vi "Plugin Configuration.Create.vi"(8 "error in (no error)":errorcluster, 10 "Plugin Configuration cluster":T1={"name"="", "class"="", "cycle timing"={"priority"=0, "decimation"=1, "offset"=0}, "Transfer Groups"=[], "settings"=[]}, 11 "Plugin Configuration in":refnum<class "Plugin Configuration.lvclass">) -> (0 "error out":errorcluster, 3 "Plugin Configuration out":refnum<class "Plugin Configuration.lvclass">)   [LabVIEW 2017, in "DSF Core.lvlib" / "Plugin Configuration.lvclass"]
uses:
  Plugin Configuration.lvclass
  DSF Configuration API/Public/Controls/DSF Engine Plugin Configuration.ctl
  DSF Configuration API/Public/Controls/DSF Timing Info.ctl
  DSF Configuration API/Public/Controls/DSF Engine Transfer Group Configuration.ctl
  DSF Configuration API/Public/Controls/DSF Direction.ctl
  DSF Configuration API/Public/Controls/DSF Engine Transfer Configuration.ctl
  DSF Configuration API/Public/Controls/DSF Byte Order.ctl
  DSF Configuration API/Public/Controls/DSF Engine Channel Configuration.ctl
  DSF Configuration API/Public/Controls/DSF Data Type.ctl
  DSF Configuration API/Public/Controls/DSF Settings Info.ctl
  Transfer Group/Transfer Group Configuration.lvclass
  Plugin Configuration.lvclass/Plugin Configuration.ctl
  DSF Core.lvlib
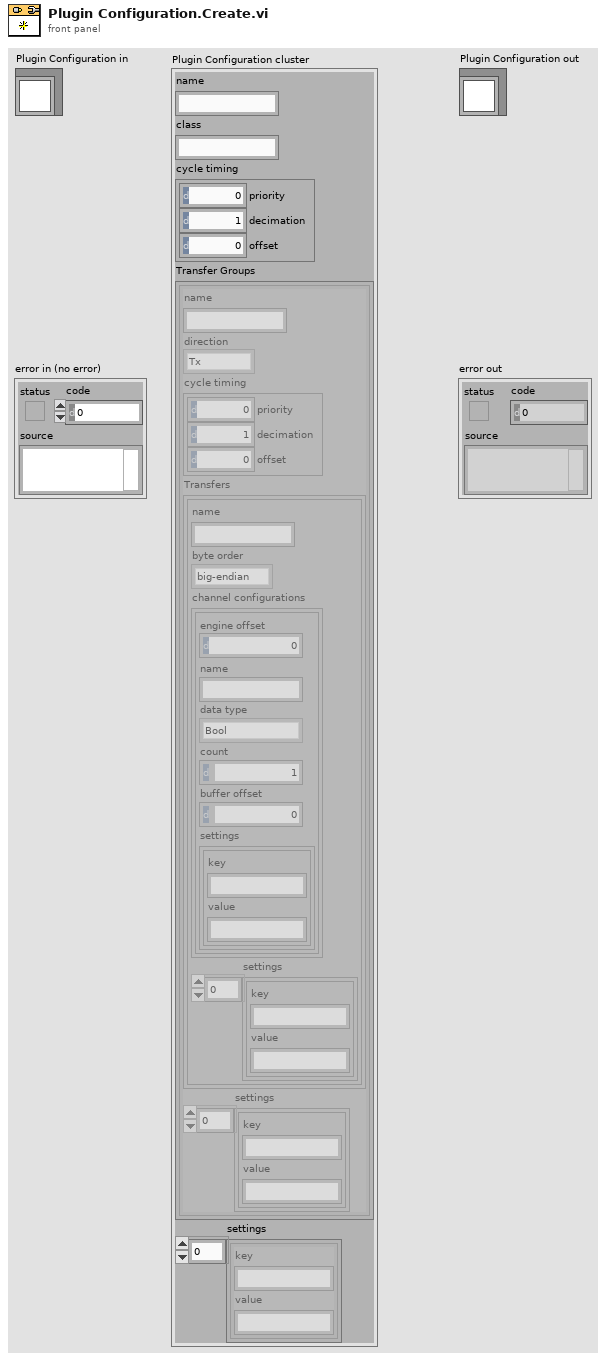
[diagram p1: front panel]
types:
  T1 = typedef "DSF Core.lvlib/DSF Engine Plugin Configuration.ctl" = cluster{"name":string, "class":string, "cycle timing":T2, "Transfer Groups":T3[], "settings":T9}
  T2 = typedef "DSF Core.lvlib/DSF Timing Info.ctl" = cluster{"priority":u64, "decimation":u64, "offset":u64}
  T3 = typedef "DSF Core.lvlib/DSF Engine Transfer Group Configuration.ctl" = cluster{"name":string, "direction":T4, "cycle timing":T2, "Transfers":T5[], "settings":T9}
  T4 = typedef "DSF Core.lvlib/DSF Direction.ctl" = enum8{"Tx", "Rx"}
  T5 = typedef "DSF Core.lvlib/DSF Engine Transfer Configuration.ctl" = cluster{"name":string, "byte order":T6, "channel configurations":T7[], "settings":T9}
  T6 = typedef "DSF Core.lvlib/DSF Byte Order.ctl" = enum8{"big-endian", "little-endian"}
  T7 = typedef "DSF Core.lvlib/DSF Engine Channel Configuration.ctl" = cluster{"engine offset":u64, "name":string, "data type":T8, "count":u64, "buffer offset":u64, "settings":T9}
  T8 = typedef "DSF Core.lvlib/DSF Data Type.ctl" = enum8{"Bool", "SGL", "DBL", "I8", "I16", "I32", "I64", "U8", "U16", "U32", "U64"}
  T9 = typedef "DSF Core.lvlib/DSF Settings Info.ctl" = cluster{"key":string, "value":string}[]
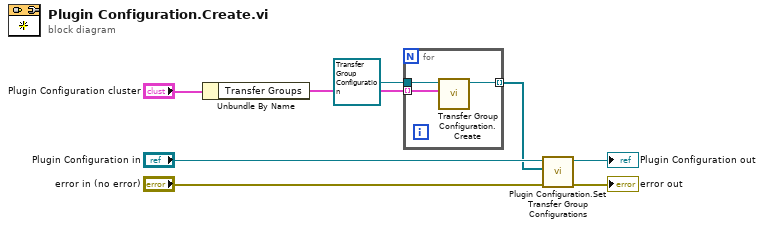
[diagram p0: block diagram]
diagram:
  n1 = Unbundle By Name("Plugin Configuration cluster") -> ("Transfer Groups"=w3:T3[])
  n2 = for {
    tunnel: w3 -> [w10] mode=indexing
    tunnel: refnum<class "Transfer Group Configuration.lvclass"> refnum ("DSF.Shared.lvlib:Transfer Group Configuration") -> [w9]
    tunnel: [w8] -> w1 mode=indexing
    n3 = call "Transfer Group Configuration.Create.vi"("Transfer Group Configuration"=w10, "Transfer Group Configuration in"=w9) -> ("Transfer Group Configuration out"=w8:refnum<class "Transfer Group Configuration.lvclass">)  [unwired: 8 in, 1 out]
  }
  n4 = call "Plugin Configuration.Set Transfer Group Configurations.vi"("Transfer Group Configurations"=w1, "Plugin Configuration in"="Plugin Configuration in") -> ("Plugin Configuration out"=→"Plugin Configuration out":refnum<class "Plugin Configuration.lvclass">)  [unwired: 9 in]
  "error out" <- "error in (no error)"
